vi "pointer.allocate empty byte array.vi"(8 "error in (no error)":errorcluster, 11 "Pointer in":refnum<class "Memory.Pointer.lvclass">) -> (0 "error out":errorcluster, 2 "empty byte array":u8[](array[numeric]), 3 "Pointer out":refnum<class "Memory.Pointer.lvclass">)   [LabVIEW 2016, in "TestCase.Pointer.lvclass"]
uses:
  TestCase.Pointer.lvclass
  Source/Classes/Pointer/Memory.Pointer.lvclass
  Source/Classes/Pointer/Memory.Pointer.lvclass/Memory.Pointer.ctl
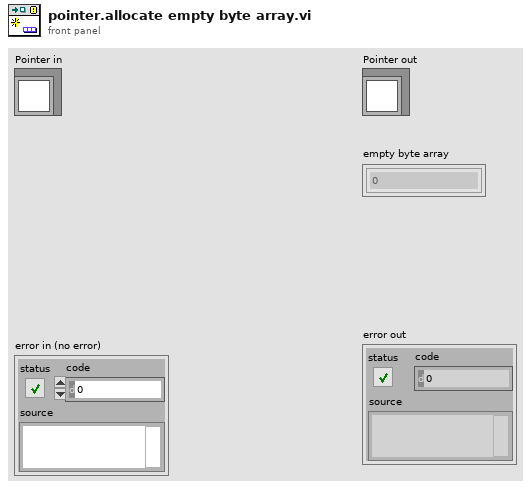
[diagram p1: front panel]
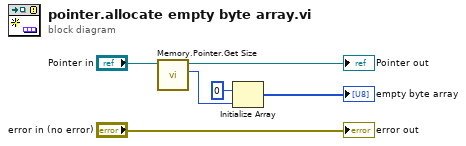
[diagram p0: block diagram]
diagram:
  n1 = call "Memory.Pointer.Get Size.vi"("Pointer in"="Pointer in") -> ("size"=w4:u64, "Pointer out"=→"Pointer out":refnum<class "Memory.Pointer.lvclass">)  [unwired: 9 in]
  n2 = Initialize Array(u8 0 ("element"), w4) -> (→"empty byte array":u8[])
  "error out" <- "error in (no error)"
